vi "Autofocus Finish.vi"(8 "error in (no error)":errorcluster, 11 "Stage Controller in":refnum<class "Stage Controller.lvclass">) -> (0 "error out":errorcluster, 3 "Stage Controller out":refnum<class "Stage Controller.lvclass">)   [LabVIEW 2023, in "Stage Controller.lvlib" / "Stage Controller.lvclass"]
uses:
  Stage Controller.lvclass
  Stage Controller.lvclass/Stage Controller.ctl
  <vilib>/Analysis/NI_AALPro.lvlib
  Microscope/ti2lv/ti2lv.lvlib
panel:
  out "center":dbl
  out "standard deviation":dbl
  out "Best Gaussian Fit":dbl[](array[numeric]) format="%#.2f"
  out "Autofocus Z":dbl[](array[numeric])
  out "Brenner Gradient":dbl[](array[numeric])
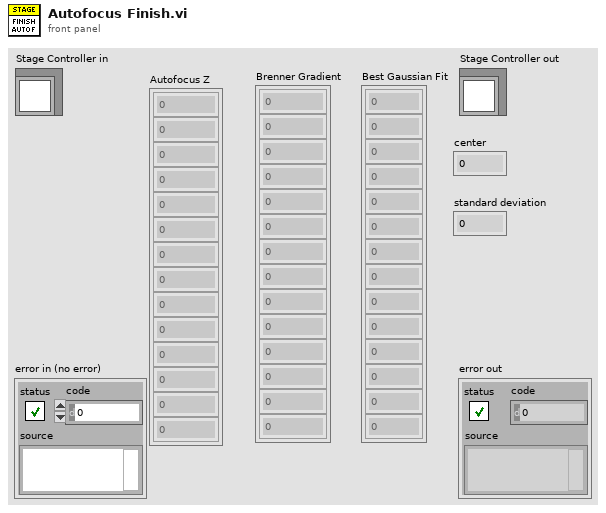
[diagram p1: front panel]
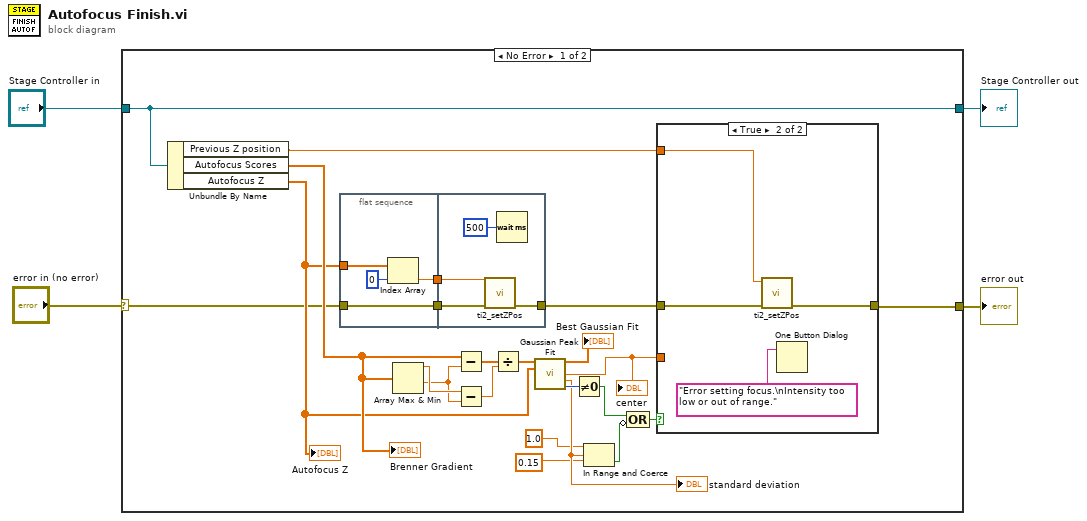
[diagram p0: block diagram]
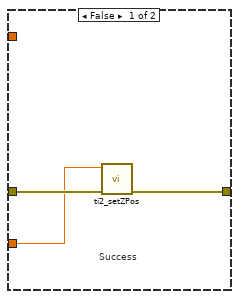
[diagram p2: hidden frame]
diagram:
  n1 = case shown="No Error" "error in (no error)" {
    selector: "error in (no error)" -> [w6 w44]
    tunnel: [w23 w44] -> w3
    tunnel: [w9 w43] -> w1
    tunnel: "Stage Controller in" -> [w9 w43]
    frame No Error {
      n2 = Unbundle By Name(w9) -> ("Previous Z position"=w5:dbl, "Autofocus Scores"=w19:dbl[], "Autofocus Z"=w7:dbl[])
      "Brenner Gradient" <- w19
      "Autofocus Z" <- w7
      n3 = flat-sequence "Move down first to ensure motor is engaged" {
        tunnel: w6 -> [w31]
        tunnel: [w31] -> w10
        tunnel: w7 -> [w30]
        tunnel: [w29] -> w8
        tunnel: [w33] -> w25
        tunnel: w10 -> [w34]
        tunnel: w8 -> [w32]
        frame #0 {
          n4 = Index Array(array=w30, index=0) -> (element=w29:dbl)
        }
        frame #1 {
          n5 = call "ti2_setZPos.vi"("error in (no error)"=w34, "z Position (um)"=w32) -> ("error out"=w33:errorcluster)  [unwired: 9 in]
          n6 = Wait (ms)(milliseconds to wait=u32 500) -> ()  [unwired: 1 out]
        }
      }
      n7 = Array Max & Min(array=w19) -> (max value=w16:dbl, min value=w15:dbl)  [unwired: 2 out]
      n8 = Subtract(x=w19, y=w15) -> (x-y=w18:dbl[])
      n9 = Subtract(x=w16, y=w15) -> (x-y=w17:dbl)
      n10 = Divide(x=w18, y=w17) -> (x/y=w27:dbl[])
      n11 = call <vilib>:"Gaussian Peak Fit.vi"("Y"=w27, "X"=w7) -> ("Best Gaussian Fit"=→"Best Gaussian Fit":dbl[], "center"=w24:dbl, "standard deviation"=w14:dbl, "error"=w26:i32)  [unwired: 7 in, 3 out]
      "standard deviation" <- w14
      "center" <- w24
      n12 = Not Equal To 0?(x=w26) -> (x != 0?=w20:bool)
      n13 = In Range and Coerce(upper limit=1.0, x=w14, lower limit=0.15) -> (In Range?=w13:bool)  [unwired: 1 out]
      n14 = Compound Arithmetic op=OR(w20, invert w13) -> (w21:bool)
      n15 = case shown="True" w21 {
        tunnel: w25 -> [w37 w41]
        tunnel: w24 -> [w36 _]
        tunnel: [w38 w40] -> w23
        tunnel: w5 -> [_ w39]
        frame False {
          # "Success"
          n16 = call "ti2_setZPos.vi"("error in (no error)"=w37, "z Position (um)"=w36) -> ("error out"=w38:errorcluster)  [unwired: 9 in]
        }
        frame True {
          n17 = call "ti2_setZPos.vi"("error in (no error)"=w41, "z Position (um)"=w39) -> ("error out"=w40:errorcluster)  [unwired: 9 in]
          n18 = One Button Dialog(message="Error setting focus.\nIntensity too low or out of range.") -> ()  [unwired: 1 in, 1 out]
        }
      }
    }
    frame Error {
    }
  }
  "error out" <- w3
  "Stage Controller out" <- w1
